vi "Rd Wr settings json CryoServer Channels.vi"(8 "error in (no error)":errorcluster, 9 "Settings File":string="CC CryoServer Log Settings.json", 10 "Write? (F:Read)":bool, 11 "CryoServer Channels":map{string, T1}(c390)) -> (0 "error out":errorcluster, 2 "Ch Names":string[][](array[string]), 3 "CryoServer Channels out":map{string, T1}(c390))   [LabVIEW 2021]
uses:
  CryoServer Channel Mapping.ctl
  2e80df6d-94aa-46b9-8b94-ceea8c057880.vi
  659fb017-0e9f-42f9-b06e-930303f00cbc.vi
  <vilib>/JDP Science/JSONtext/Find Item.vi
  <vilib>/JDP Science/JSONtext/Next JSON Value.vi
  <vilib>/JDP Science/JSONtext/String Subset.vi
  <vilib>/JDP Science/JSONtext/Parsing/Advance past next JSON Value (inlined COPY).vi
  <vilib>/JDP Science/JSONtext/Parsing/Advance past whitespace.vi
  <vilib>/JDP Science/JSONtext/Parsing/Advance past String.vi
  <vilib>/JDP Science/JSONtext/Parsing/Advance past Number.vi
  <vilib>/JDP Science/JSONtext/Parsing/Advance past Line Ending.vi
  <vilib>/JDP Science/JSONtext/Parsing/Parse Full Path or Item Name.vi
  <vilib>/JDP Science/JSONtext/Parsing/Advance past Array.vi
  <vilib>/JDP Science/JSONtext/Parsing/Advance past Object.vi
  <vilib>/JDP Science/JSONtext/support/Error Cluster From Code.vi
  <vilib>/JDP Science/JSONtext/Offset/Find Item Locations by Path.vi
  <vilib>/JDP Science/JSONtext/JSON text to Variant.vi
  <vilib>/JDP Science/JSONtext/Variant to JSON Text.vi
  <vilib>/JDP Science/JSONtext/Set Item.vi
  <vilib>/JDP Science/JSONtext/LVClass Serializer/JSONtext LVClass Serializer.lvclass
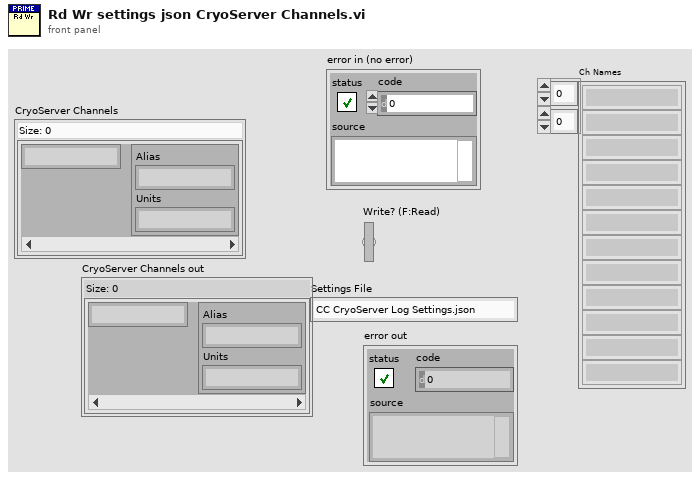
[diagram p1: front panel]
types:
  T1 = typedef "CryoServer Channel Mapping.ctl" = cluster{"Alias":string, "Units":string}
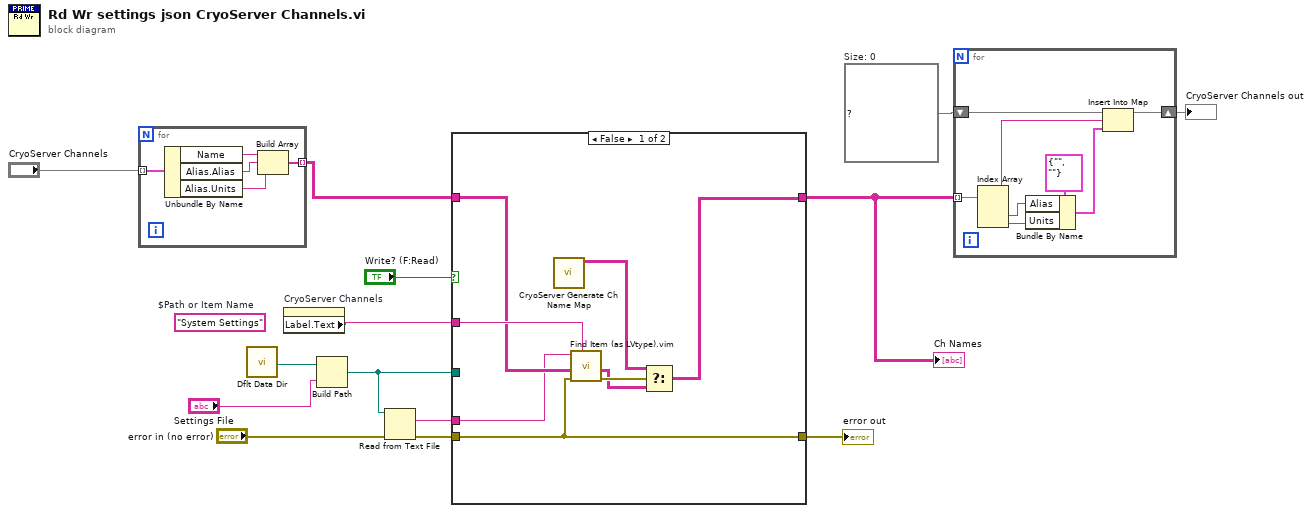
[diagram p0: block diagram]
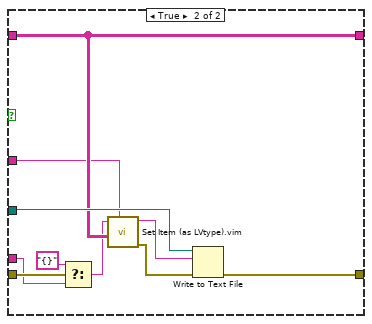
[diagram p2: hidden frame]
diagram:
  w6 = map{string, T1} {}  # Size: 0
  (unwired) "System Settings"  # $Path or Item Name
  n1 = for {
    tunnel: "CryoServer Channels" -> [w19] mode=indexing
    tunnel: [w15] -> w3 mode=indexing
    n2 = Unbundle By Name(w19) -> ("Name"=w18:string, "Alias.Alias"=w17:string, "Alias.Units"=w16:string)
    n3 = Build Array(w18, w17, w16) -> (w15:string[])
  }
  n4 = call <vilib>:"Dflt Data Dir.vi"() -> ("App:Default Data Directory"=w12:path)
  n5 = property on="CryoServer Channels" class="Map (strict)"() -> ("Label.Text"=w4:string)  [unwired: 2 in, 2 out]
  n6 = Build Path(base path=w12, name or relative path="Settings File") -> (appended path=w7:path)
  n7 = Read from Text File(file (use dialog)=w7, error in="error in (no error)") -> (text=w8:string, error out=w9:errorcluster)  [unwired: 2 in, 2 out]
  n8 = case shown="False" "Write? (F:Read)" {
    tunnel: w9 -> [w21 w32]
    tunnel: w3 -> [w25 w35]
    tunnel: w7 -> [_ w37]
    tunnel: [w21 w36] -> w11
    tunnel: [w27 w35] -> w2
    tunnel: w4 -> [w26 w34]
    tunnel: w8 -> [w22 w30]
    frame False {
      n9 = call "CryoServer Generate Ch Name Map.vi"() -> ("Generate Table"=w20:string[][])  [unwired: 11 in]
      n10 = call "Find Item (as LVtype).vim"("$Path or Item Name"=w26, "error in (no error)"=w21, "Data Type and Default Value"=w25, "JSON"=w22) -> ("error out"=w24:errorcluster, "Data"=w23:string[][])  [unwired: 4 in, 2 out]
      n11 = Select(t=w20, s=w24, f=w23) -> (s? t:f=w27:string[][])
    }
    frame True {
      n12 = Select(t="{}" ("JSON"), s=w32, f=w30) -> (s? t:f=w29:string)
      n13 = call "Set Item (as LVtype).vim"("$Path or Item Name"=w34, "Anything"=w35, "JSON"=w29) -> ("error out"=w28:errorcluster, "<JSON>"=w33:string)  [unwired: 5 in, 1 out]
      n14 = Write to Text File(file (use dialog)=w37, text=w33, error in=w28) -> (error out=w36:errorcluster)  [unwired: 1 in, 2 out]
    }
  }
  "error out" <- w11
  "Ch Names" <- w2
  n15 = for {
    shift-right: [w43] -> w1
    shift-left: w6 -> [w45]
    tunnel: w2 -> [w41] mode=indexing
    n16 = Index Array(array=w41) -> (element #1=w38:string, element #2=w40:string, element #3=w39:string)  [unwired: 3 in]
    n17 = Bundle By Name(cluster=T1 {"Alias"="", "Units"=""} ("value"), "Alias"=w40, "Units"=w39) -> (w44:T1)
    n18 = Insert Into Map(map in=w45, key=w38, value=w44) -> (map out=w43:map{string, T1})  [unwired: 2 out]
  }
  "CryoServer Channels out" <- w1
